vi "19052 Get_instrument_ID.vi"(8 "error in":errorcluster, 11 "VISA resource name in":refnum<visa-resource-name>) -> (0 "error out":errorcluster, 2 "instrument ID":string, 3 "VISA resource name out":refnum<visa-resource-name>)   [LabVIEW 2015]
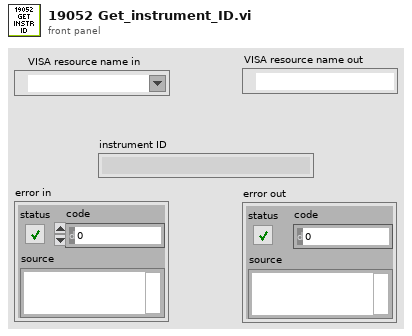
[diagram p1: front panel]
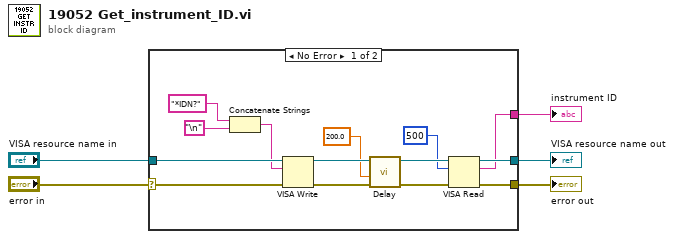
[diagram p0: block diagram]
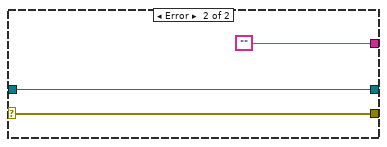
[diagram p2: hidden frame]
diagram:
  n1 = case shown="No Error" "error in" {
    selector: "error in" -> [w17 w21]
    tunnel: [w18 w21] -> w5
    tunnel: [w11 ""] -> w3
    tunnel: [w16 w19] -> w2
    tunnel: "VISA resource name in" -> [w15 w19]
    frame No Error {
      n2 = Concatenate Strings("*IDN?" ("write buffer"), "\n") -> (w12:string)
      n3 = VISA Write(VISA resource name=w15, write buffer=w12, error in (no error)=w17) -> (VISA resource name out=w8:refnum<visa-resource-name>, error out=w10:errorcluster)  [unwired: 1 out]
      n4 = call "Delay.vi"("error in (no error)"=w10, "milliseconds to wait"=200.0) -> ("error out"=w9:errorcluster)  [unwired: 9 in]
      n5 = VISA Read(VISA resource name=w8, byte count=u32 500, error in (no error)=w9) -> (VISA resource name out=w16:refnum<visa-resource-name>, read buffer=w11:string, error out=w18:errorcluster)  [unwired: 1 out]
    }
    frame Error {
    }
  }
  "error out" <- w5
  "VISA resource name out" <- w2
  "instrument ID" <- w3
